vi "Show Image Value in TipStrip.vi"(8 "error in (no error)":errorcluster, 11 "Image Display Refnum":T1 caption="Image Control Refnum") -> (0 "error out":errorcluster)   [LabVIEW 2021, in "Image.lvlib"]
doc: "Displays the (SGL) image value at the last mouse poistion in tipstrip."
uses:
  Image.lvlib
  Image Control Refnum.ctl
  <vilib>/vision/NI_Vision_Development_Module.lvlib
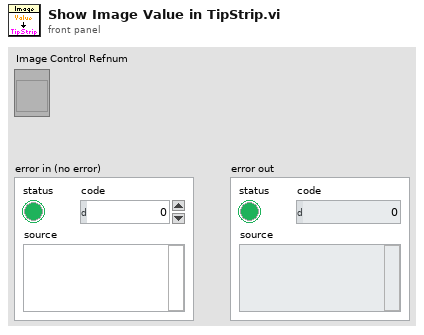
[diagram p1: front panel]
types:
  T1 = typedef "Image.lvlib/Image Control Refnum.ctl" = refnum<vi>
  T2 = typedef "IMAQ Image.ctl" = refnum<image>
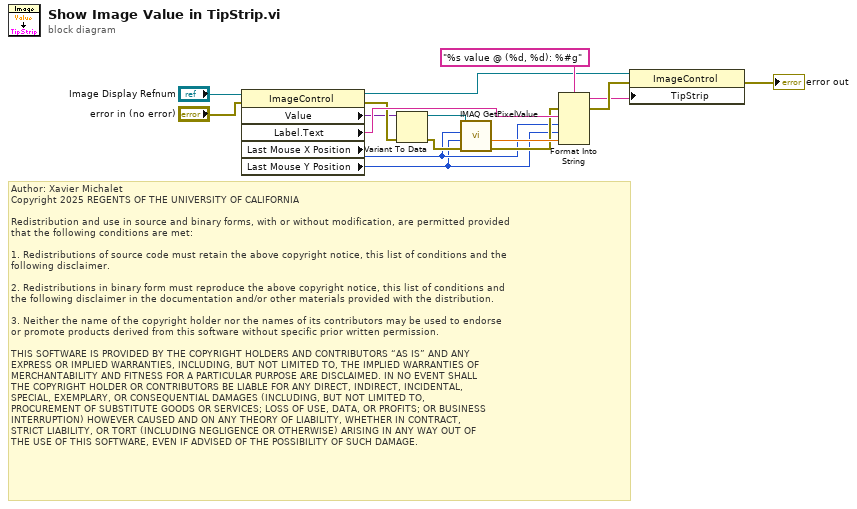
[diagram p0: block diagram]
diagram:
  # "Author: Xavier Michalet\nCopyright 2025 REGENTS OF THE UNIVERSITY OF CALIFORNIA\n\nRedistribution and use in source and binary forms, with or without modification, are permitted provided\nthat the following conditions are met:\n\n1. Redistributions of source code must retain the above copyright notice, this list of conditions and the\nfollowing disclaimer.\n\n2. Redistributions in binary form must reproduce the above copyright notice, this list of conditions and\nthe following disclaimer in the documentation and/or other materials provided with the distribution.\n\n3. Neither the name of the copyright holder nor the names of its contributors may be used to endorse \nor promote products derived from this software without specific prior written permission.\n\nTHIS SOFTWARE IS PROVIDED BY THE COPYRIGHT HOLDERS AND CONTRIBUTORS “AS IS” AND ANY \nEXPRESS OR IMPLIED WARRANTIES, INCLUDING, BUT NOT LIMITED TO, THE IMPLIED WARRANTIES OF\nMERCHANTABILITY AND FITNESS FOR A PARTICULAR PURPOSE ARE DISCLAIMED. IN NO EVENT SHALL\nTHE COPYRIGHT HOLDER OR CONTRIBUTORS BE LIABLE FOR ANY DIRECT, INDIRECT, INCIDENTAL, \nSPECIAL, EXEMPLARY, OR CONSEQUENTIAL DAMAGES (INCLUDING, BUT NOT LIMITED TO, \nPROCUREMENT OF SUBSTITUTE GOODS OR SERVICES; LOSS OF USE, DATA, OR PROFITS; OR BUSINESS\nINTERRUPTION) HOWEVER CAUSED AND ON ANY THEORY OF LIABILITY, WHETHER IN CONTRACT, \nSTRICT LIABILITY, OR TORT (INCLUDING NEGLIGENCE OR OTHERWISE) ARISING IN ANY WAY OUT OF\nTHE USE OF THIS SOFTWARE, EVEN IF ADVISED OF THE POSSIBILITY OF SUCH DAMAGE."
  n1 = property class="ImageControl"(reference="Image Display Refnum", error in="error in (no error)") -> (reference out=w8:T1, error out=w6:errorcluster, "Value"=w4:variant, "Label.Text"=w16:string, "Last Mouse X Position"=w2:i32, "Last Mouse Y Position"=w1:i32)
  n2 = Variant To Data(error in=w6, Variant=w4) -> (data=w5:T2, error out=w7:errorcluster)  [unwired: 1 in]
  n3 = call "IMAQ GetPixelValue"("Image"=w5, "X Coordinate"=w2, "Y Coordinate"=w1, "error in (no error)"=w7) -> ("Pixel Value (Float)"=w15:sgl, "error out"=w11:errorcluster)  [unwired: 2 in, 3 out]
  n4 = Format Into String(format string="%s value @ (%d, %d): %#g", error in=w11, w16, w2, w1, w15) -> (resulting string=w10:string, error out=w12:errorcluster)  [unwired: 1 in]
  n5 = property class="ImageControl"(reference=w8, error in=w12, "TipStrip"=w10) -> (error out=→"error out":errorcluster)  [unwired: 1 out]
